vi "RPM 800 速度轉電壓 三軸平台 Axis 1.vi"(1 "Speed (1mm/s)":dbl) -> (0 "Voltage\nOutput":dbl)   [LabVIEW 2019]
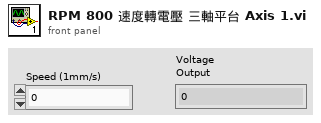
[diagram p1: front panel]
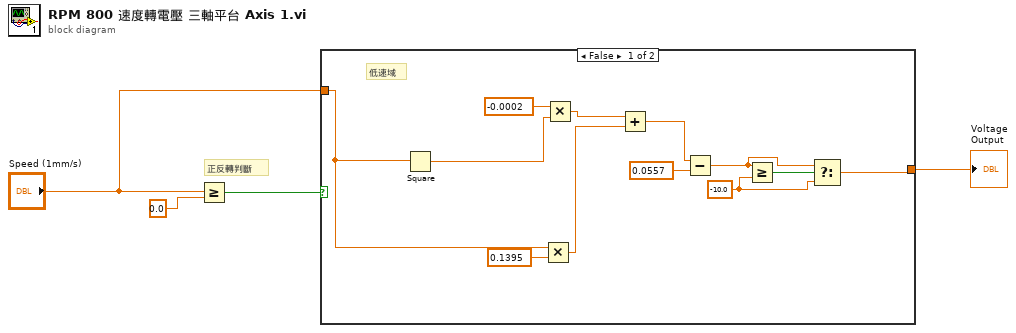
[diagram p0: block diagram]
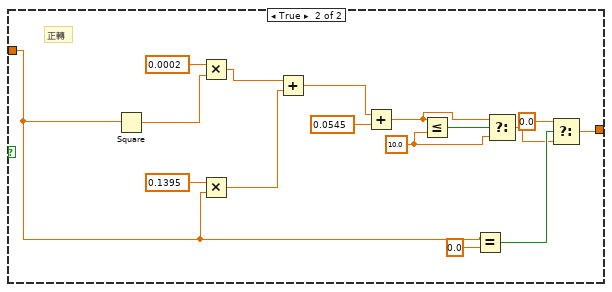
[diagram p2: hidden frame]
diagram:
  # "正反轉判斷"
  n1 = Greater Or Equal?(x="Speed (1mm/s)", y=0.0) -> (x >= y?=w3:bool)
  n2 = case shown="False" w3 {
    tunnel: "Speed (1mm/s)" -> [w6 w22]
    tunnel: [w8 w20] -> w1
    frame False {
      w10 = -10.0 ("y")
      # "低速域"
      n3 = Square(x=w6) -> (x^2=w16:dbl)
      n4 = Multiply(x=w6, y=0.1395) -> (x*y=w12:dbl)
      n5 = Multiply(x=-0.0002, y=w16) -> (x*y=w15:dbl)
      n6 = Add(x=w15, y=w12) -> (x+y=w14:dbl)
      n7 = Subtract(x=w14, y=0.0557) -> (x-y=w9:dbl)
      n8 = Greater Or Equal?(x=w9, y=w10) -> (x >= y?=w11:bool)
      n9 = Select(t=w9, s=w11, f=w10) -> (s? t:f=w8:dbl)
    }
    frame True {
      w26 = 10.0 ("y")
      # "正轉"
      n10 = Square(x=w22) -> (x^2=w32:dbl)
      n11 = Multiply(x=0.0002, y=w32) -> (x*y=w31:dbl)
      n12 = Multiply(x=0.1395, y=w22) -> (x*y=w30:dbl)
      n13 = Add(x=w31, y=w30) -> (x+y=w29:dbl)
      n14 = Add(x=w29, y=0.0545) -> (x+y=w25:dbl)
      n15 = Less Or Equal?(x=w25, y=w26) -> (x <= y?=w27:bool)
      n16 = Equal?(x=w22, y=0.0) -> (x = y?=w19:bool)
      n17 = Select(t=w25, s=w27, f=w26) -> (s? t:f=w18:dbl)
      n18 = Select(t=0.0, s=w19, f=w18) -> (s? t:f=w20:dbl)
    }
  }
  "Voltage\nOutput" <- w1
